vi "PUMP_main.vi"   [LabVIEW 2015]
uses:
  CONTROLS/Q_main_element.ctl
  CONTROLS/Q_PUMP_element.ctl
  <userlib>/Fluigent/Fluigent MFCS/FluigentMFCS_Full.llb/_EZmfcsRefNum.ctl
  <userlib>/Fluigent/Fluigent MFCS/FluigentMFCS_Full.llb/_EZmfcsEnum.ctl
  <userlib>/Fluigent/Fluigent FRP/FluigentFRP.llb/_frpEnum.ctl
  <userlib>/Fluigent/Fluigent MFCS/FluigentMFCS_Full.llb/_EZmfcsSN.ctl
  GLOBAL/Global_PUMP.vi
  GLOBAL/Global_ABORT.vi
  GLOBAL/Global_MAIN.vi
  <userlib>/Fluigent/Fluigent MFCS/FluigentMFCS_Full.llb/MFCS_EZ Initialization.vi
  <userlib>/Fluigent/Fluigent MFCS/FluigentMFCS_Full.llb/MFCS_EZ Close.vi
types:
  T1 = typedef "_frpRefNum" = refnum<k1>
  T2 = typedef "_EZmfcsRefNum.ctl" = refnum<k1>
  T3 = typedef "Q_PUMP_element.ctl" = cluster{"variant":variant, "Instruction":enum16{"PUMP_idle", "PUMP_initialize", "PUMP_error", "PUMP_security_stop", "PUMP_read_pressure", "PUMP_change_pressure", "PUMP_init_merFISH", "PUMP_change_presure_merFISH", "PUMP_zero_pressure_merFISH", "PUMP_close_merFISH", "PUMP_stop"}}
  T4 = typedef "Q_main_element.ctl" = cluster{"variant":variant, "Instruction":enum16{"Main_idle", "Main_initialize", "Main_initialize_TDMS", "Main_initialize_Queue", "Main_error", "Main_DAQ_initialization_results", "Main_ASI_initialization_results", "Main_Piezo_initialization_results", "Main_Valve_initialization_results", "Main_Pump_initialization_results", "Main_CAMERA_initialization_results", "Main_FPGA_initialization_results", "Main_DAQ_error", "Main_ASI_error", "Main_Piezo_error", "Main_CAMERA_error", "Main_Valve_error", "Main_Pump_error", "Main_FPGA_error", "Main_start_acquiring", "Main_not_acquiring", "Main_acquiring", "Main_stop_acquiring", "Main_change_exposure", "Main_change_z_scan_parameters", "Main_define_ROI", "Main_define_mosaic", "Main_read_kinetic_time", "Main_cooler", "Main_read_temperature", "Main_save_XY", "Main_load_XY", "Main_discard_XY", "Main_move_to_XY", "Main_measure_QPD", "Main_autofocus_calibration", "Main_autofocus_initialization", "Main_autofocus_stop", "Main_save_PID", "Main_change_H_valve_position", "Main_two_way_valve", "Main_save_movie", "Main_init_single_scan", "Main_single_scan", "Main_stop_single_scan", "Main_merFISH_illumination_parameters", "Main_merFISH_buffer_probe_list", "Main_merFISH_injections_procedure", "Main_merFISH_save_setpoint", "Main_merFISH_DAPI_parameters", "Main_merFISH_Brightfield_parameters", "Main_merFISH_save_embryo_ROI", "Main_merFISH_init", "Main_merFISH_resume", "Main_merFISH_start_autofocus", "Main_merFISH_open_close_valve_merFISH", "Main_merFISH_open_close_valve_photobleaching", "Main_merFISH_hybridization", "Main_merFISH_move_to_ROI", "Main_merFISH_wait_stabilization", "Main_merFISH_move_to_REF", "Main_merFISH_scan", "Main_merFISH_photobleaching_injection", "Main_merFISH_photobleaching", "Main_merFISH_send_email", "Main_merFISH_close", "Main_STOP"}}
  T5 = typedef "_EZmfcsSN.ctl" = u16
  T6 = cluster{"Pressure (mbar)":i32, "Volume (µl)":i32, "Flow rate (ul/min) ":i32}
  T7 = enum16{"PUMP_idle", "PUMP_initialize", "PUMP_error", "PUMP_security_stop", "PUMP_read_pressure", "PUMP_change_pressure", "PUMP_init_merFISH", "PUMP_change_presure_merFISH", "PUMP_zero_pressure_merFISH", "PUMP_close_merFISH", "PUMP_stop"}
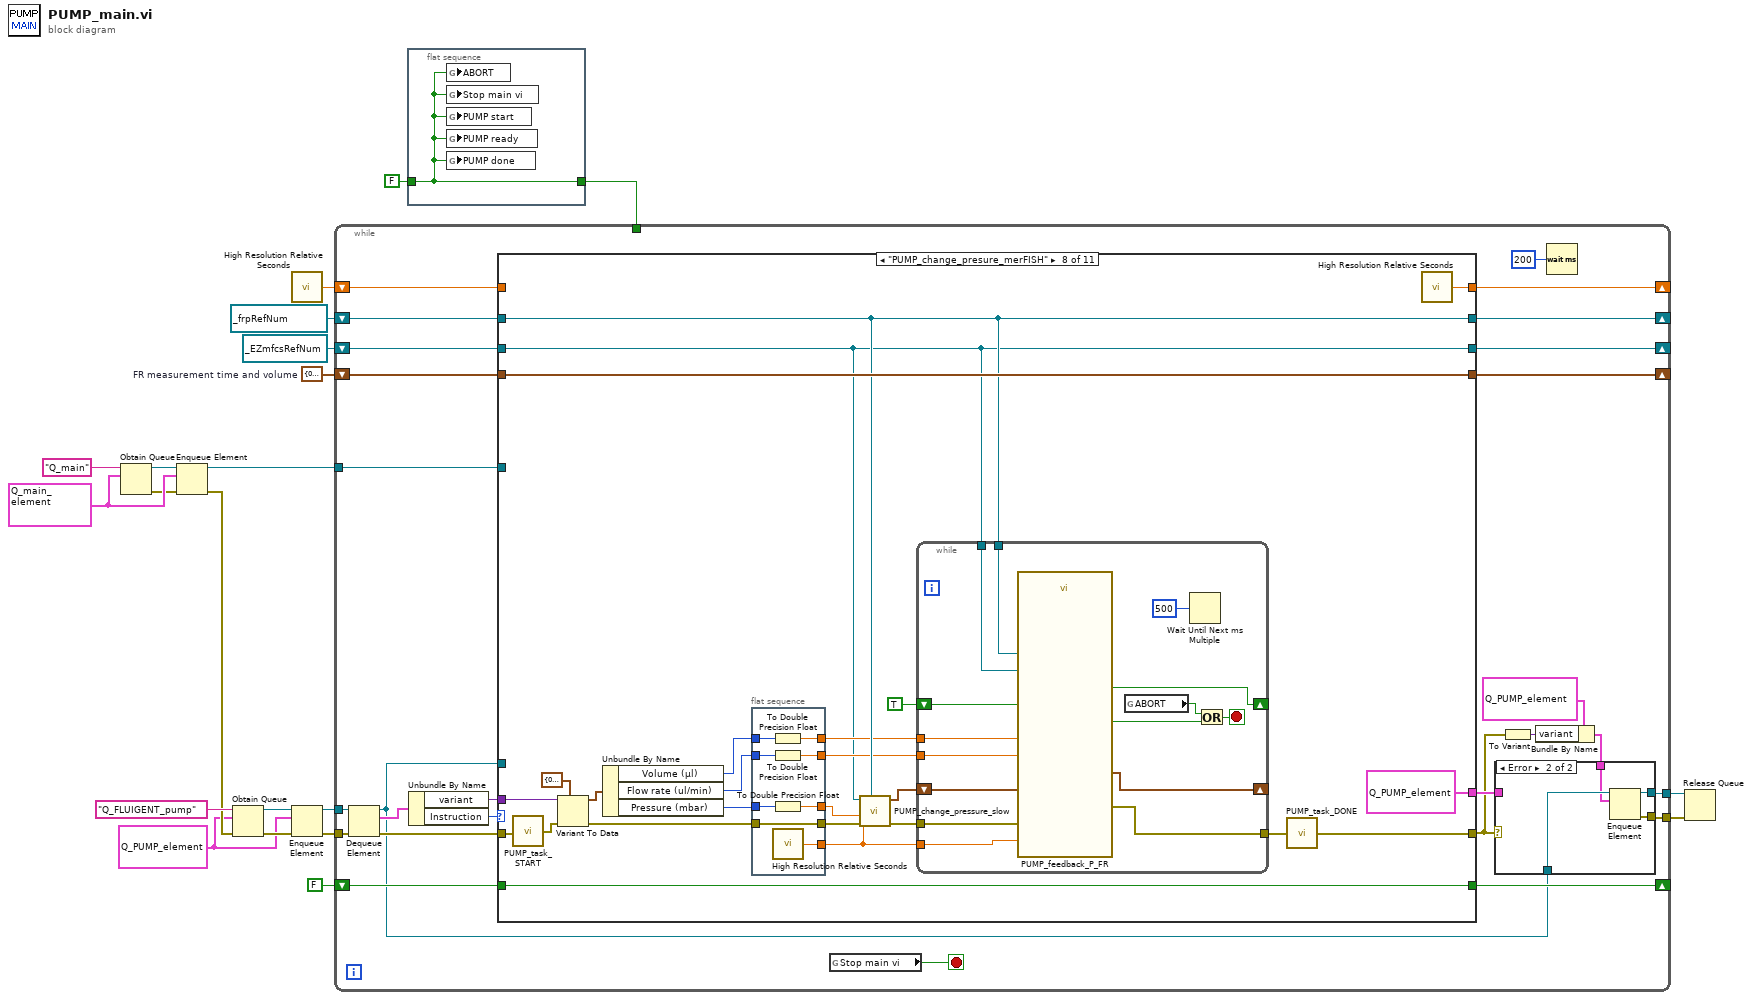
[diagram p0: block diagram]
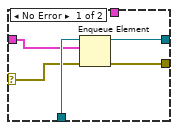
[diagram p2: hidden frame]
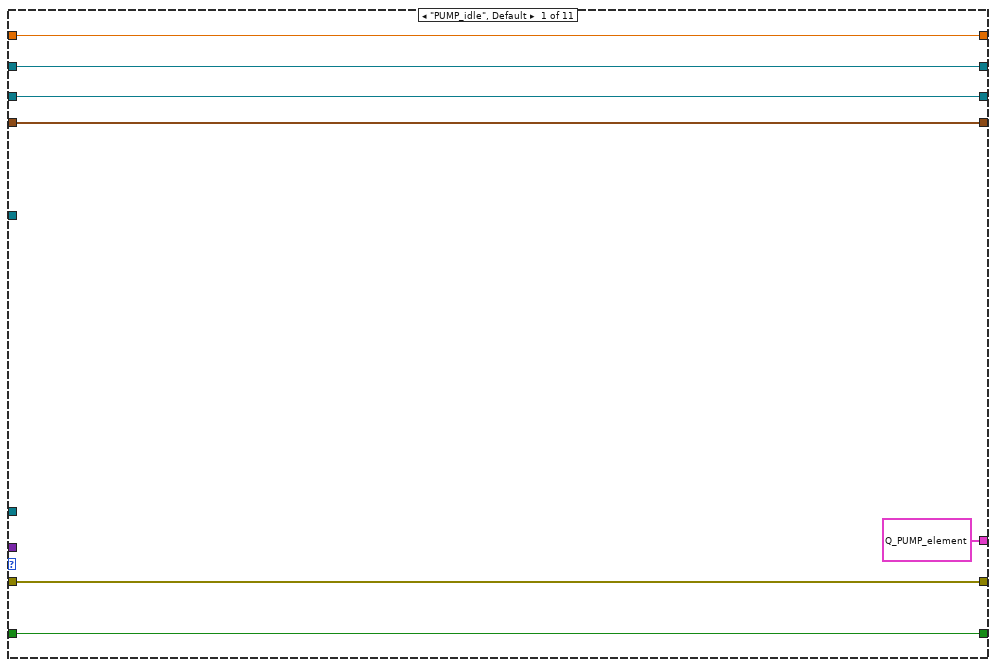
[diagram p3: hidden frame]
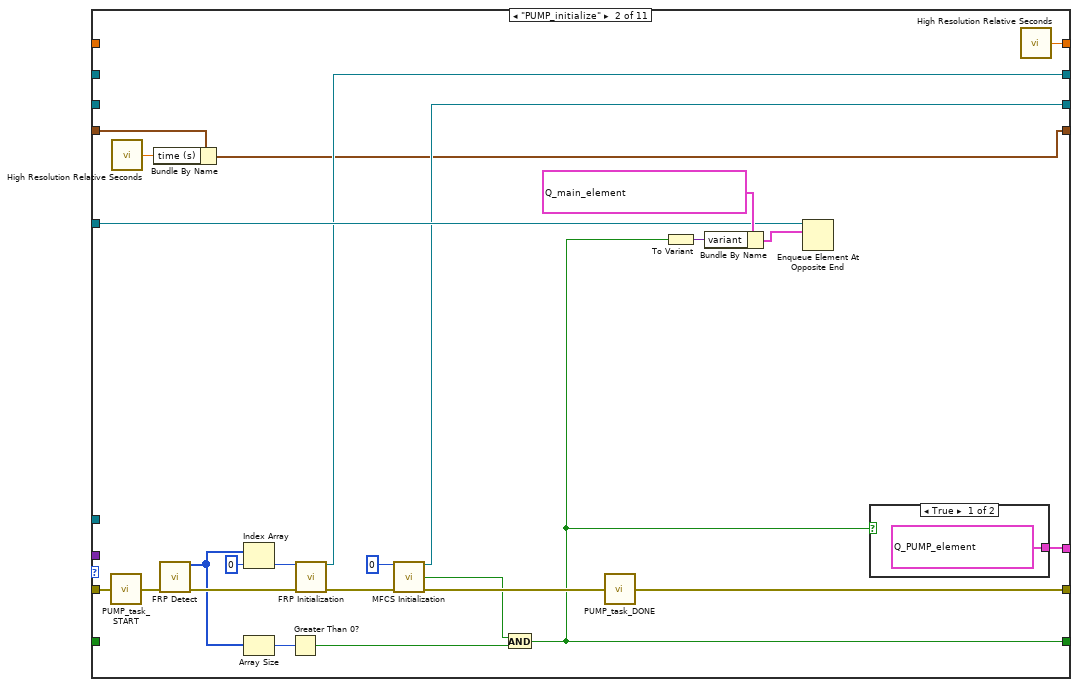
[diagram p4: hidden frame]
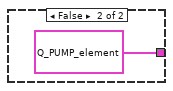
[diagram p5: hidden frame]
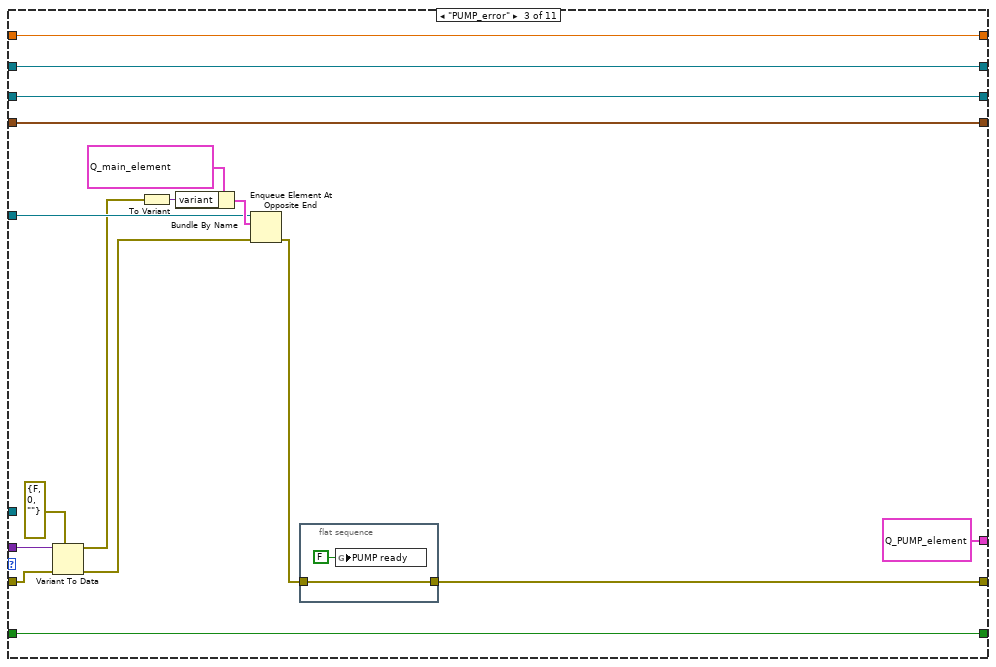
[diagram p6: hidden frame]
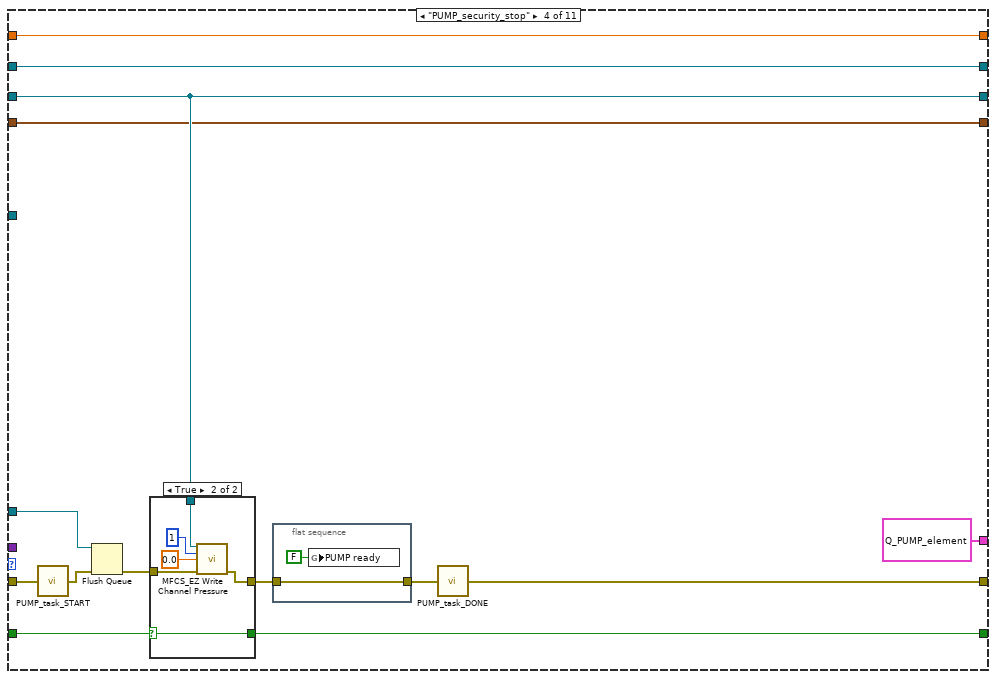
[diagram p7: hidden frame]
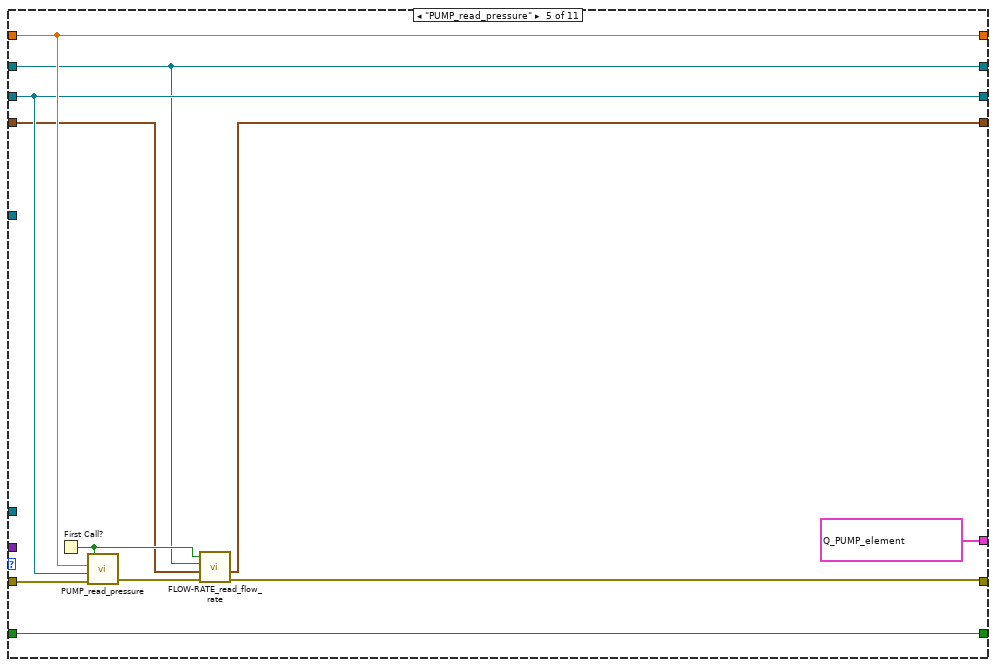
[diagram p9: hidden frame]
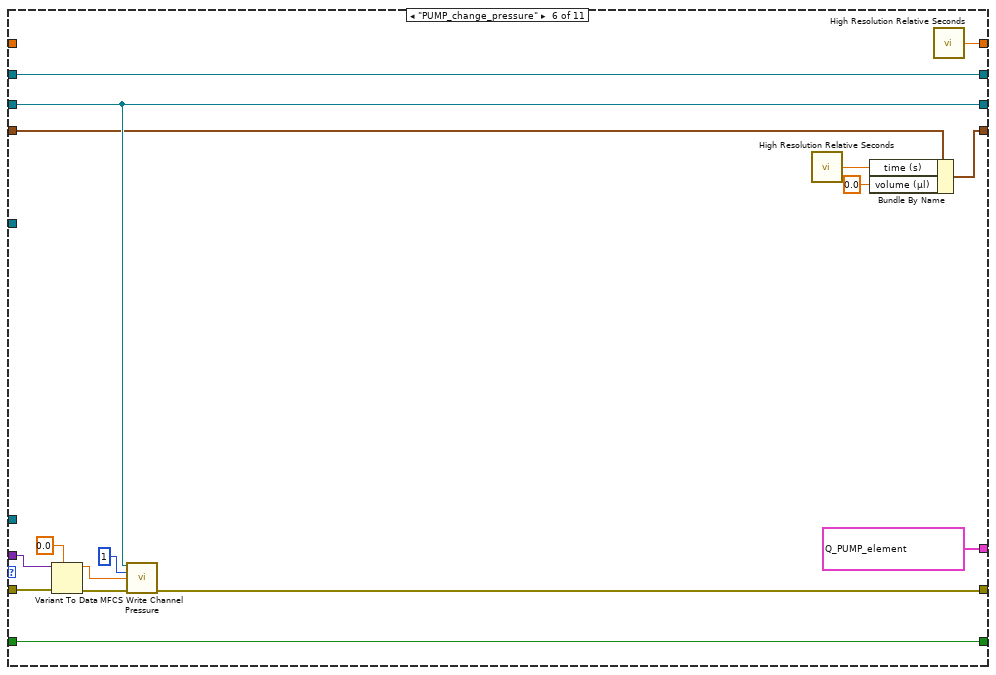
[diagram p10: hidden frame]
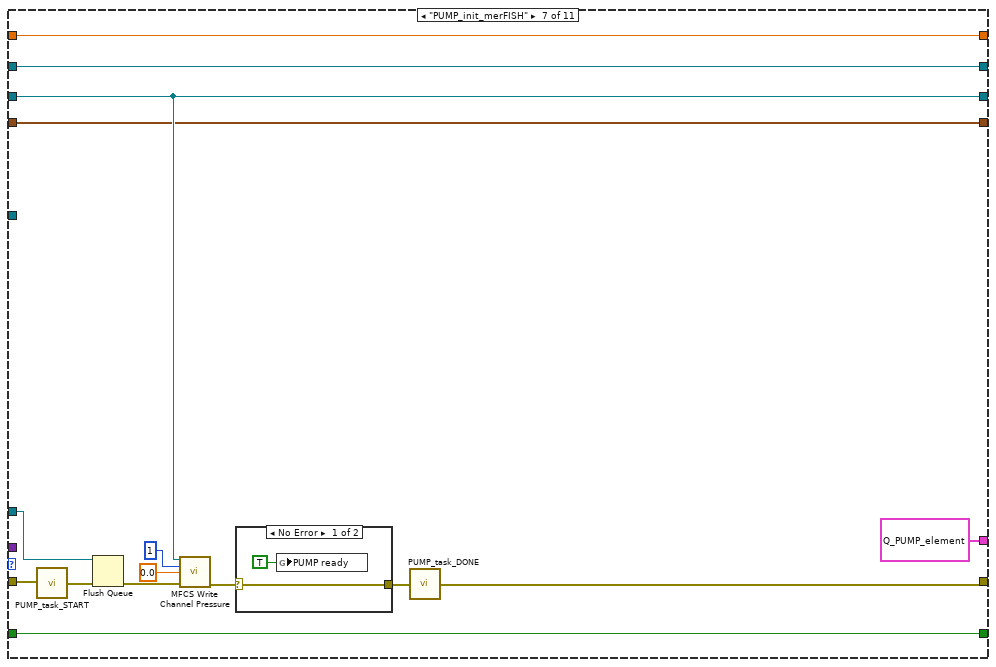
[diagram p11: hidden frame]
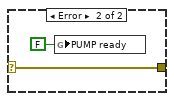
[diagram p12: hidden frame]
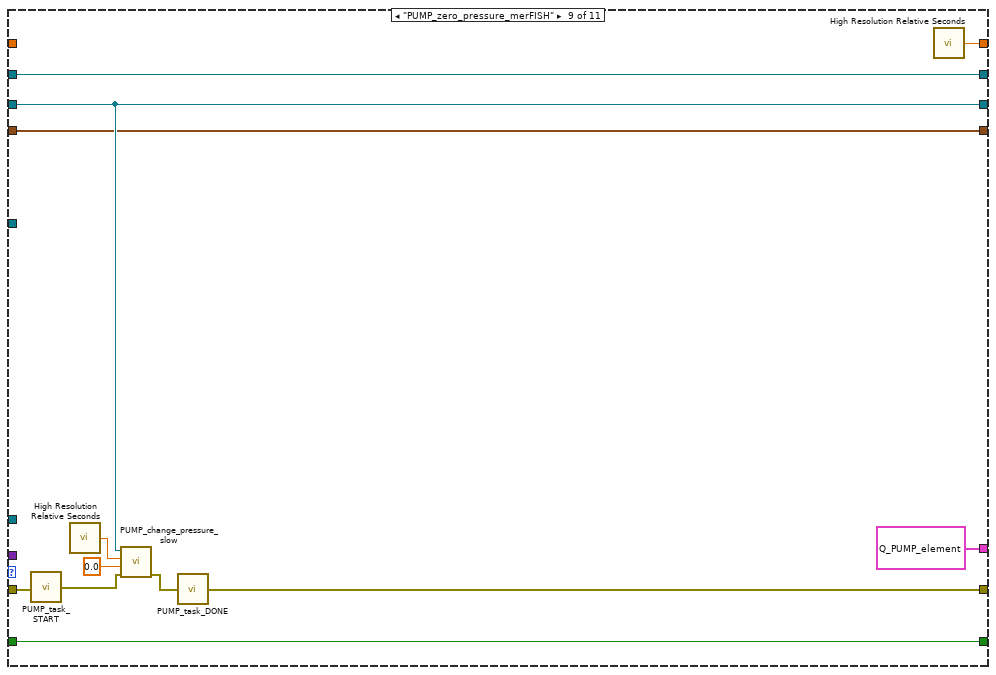
[diagram p13: hidden frame]
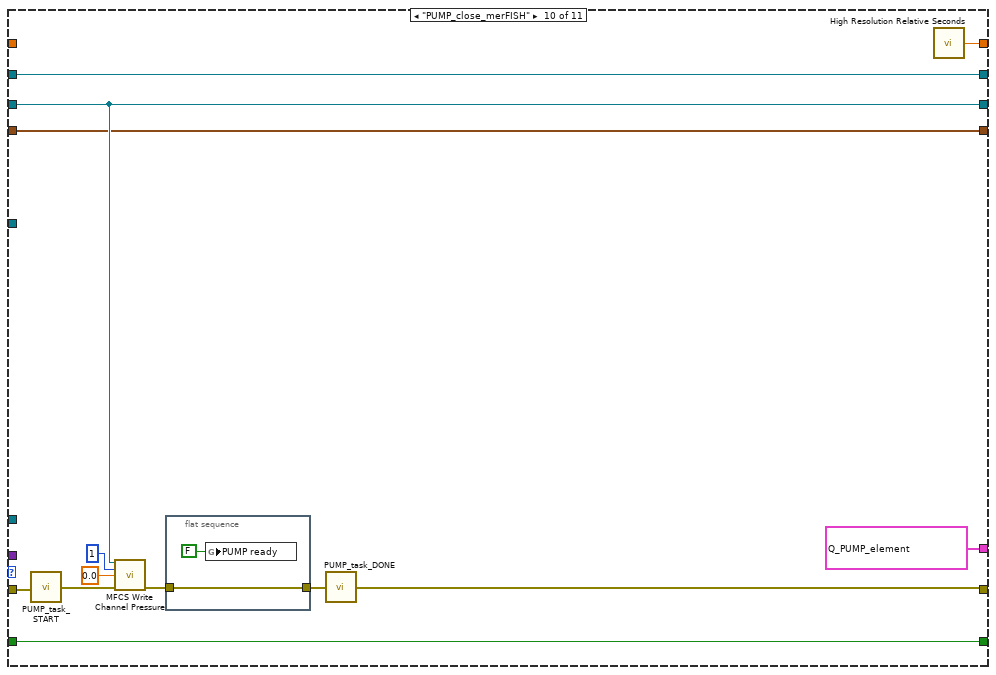
[diagram p14: hidden frame]
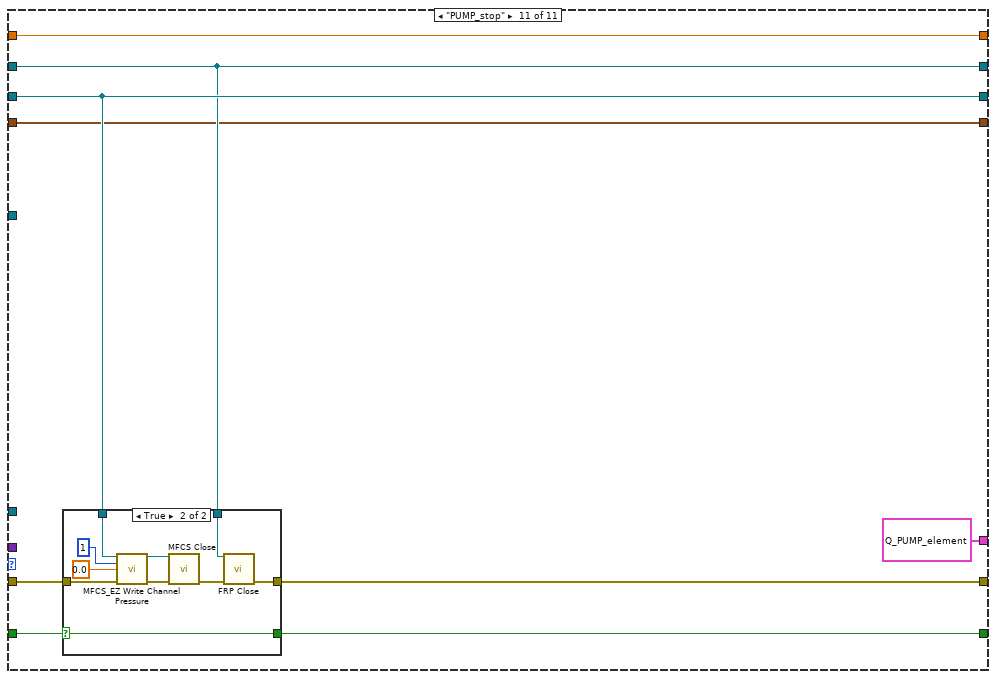
[diagram p15: hidden frame]
diagram:
  w1 = cluster{"time (s)":dbl, "volume (µl)":dbl} {"time (s)"=0.0, "volume (µl)"=0.0}  # FR measurement time and volume
  w2 = T1 refnum items=["fluigentFRP"] ("FRP out")
  w5 = T2 refnum items=["EZ_MFCS"] ("MFCS_EZ out")
  w6 = T3 {"variant"=variant, "Instruction"=enum."PUMP_idle"} ("Q_PUMP")
  w14 = T4 {"variant"=variant, "Instruction"=enum."Main_idle"} ("Q_main_element")
  n1 = Obtain Queue(name (unnamed)="Q_main", element data type=w14) -> (queue out=w12:refnum<queue>, error out=w13:errorcluster)  [unwired: 3 in, 1 out]
  n2 = Enqueue Element(queue=w12, element=w14, error in (no error)=w13) -> (queue out=w10:refnum<queue>, error out=w7:errorcluster)  [unwired: 1 in, 1 out]
  n3 = Obtain Queue(name (unnamed)="Q_FLUIGENT_pump", element data type=w6, error in (no error)=w7) -> (queue out=w20:refnum<queue>, error out=w19:errorcluster)  [unwired: 2 in, 1 out]
  n4 = call <vilib>:"High Resolution Relative Seconds.vi"() -> ("relative seconds"=w4:dbl)
  n5 = Enqueue Element(queue=w20, element=w6, error in (no error)=w19) -> (queue out=w18:refnum<queue>, error out=w17:errorcluster)  [unwired: 1 in, 1 out]
  n6 = while {
    tunnel: w18 -> [w47]
    tunnel: w17 -> [w46]
    tunnel: [w41] -> w16
    tunnel: [w40] -> w15
    tunnel: w10 -> [w39]
    tunnel: w8 -> [_]
    shift-right: [w32] -> _
    shift-left: w5 -> [w31]
    shift-right: [w30] -> _
    shift-left: w4 -> [w29]
    shift-right: [w27] -> _
    shift-left: FALSE -> [w28]
    shift-right: [w25] -> _
    shift-left: w2 -> [w26]
    shift-right: [w23] -> _
    shift-left: w1 -> [w24]
    stop <- w48 stop-if-true
    n7 = Dequeue Element(queue=w47, error in (no error)=w46) -> (queue out=w22:refnum<queue>, element=w45:T3, error out=w43:errorcluster)  [unwired: 1 in, 1 out]
    n8 = Unbundle By Name(w45) -> ("variant"=w38:variant, "Instruction"=w44:T7)
    n9 = case shown="\"PUMP_change_presure_merFISH\"" w44 {
      tunnel: w43 -> [w64 w89 w101 w123 w144 w161 w174 w201 w238 w251 w262]
      tunnel: [w64 w69 w94 w118 w140 w150 w172 w197 w237 w250 w263] -> w35
      tunnel: [T3 {"variant"=variant, "Instruction"=enum."PUMP_idle"} ("Q_PUMP") w82 T3 {"variant"=variant, "Instruction"=enum."PUMP_idle"} ("Q_PUMP") T3 {"variant"=variant, "Instruction"=enum."PUMP_idle"} ("Q_PUMP") T3 {"variant"=variant, "Instruction"=enum."PUMP_read_pressure"} ("Q_PUMP") T3 {"variant"=variant, "Instruction"=enum."PUMP_read_pressure"} ("Q_PUMP") T3 {"variant"=variant, "Instruction"=enum."PUMP_idle"} ("Q_PUMP") T3 {"variant"=variant, "Instruction"=enum."PUMP_idle"} ("Q_PUMP") T3 {"variant"=variant, "Instruction"=enum."PUMP_idle"} ("Q_PUMP") T3 {"variant"=variant, "Instruction"=enum."PUMP_read_pressure"} ("Q_PUMP") T3 {"variant"=variant, "Instruction"=enum."PUMP_idle"} ("Q_PUMP")] -> w42
      tunnel: w39 -> [_ w84 w103 _ _ _ _ _ _ _ _]
      tunnel: w38 -> [_ _ w100 _ _ w160 _ w205 _ _ _]
      tunnel: w22 -> [_ _ _ w121 _ _ w167 _ _ _ _]
      tunnel: [w62 w83 w107 w119 w138 w152 w164 w183 w236 w244 w261] -> w32
      tunnel: w31 -> [w62 _ w107 w119 w138 w152 w164 w183 w236 w244 w261]
      tunnel: [w61 w81 w97 w117 w143 w154 w176 w203 w239 w252 w260] -> w30
      tunnel: w29 -> [w61 _ w97 w117 w143 _ w176 _ _ _ w260]
      tunnel: w28 -> [w60 _ w96 w116 w142 w153 w165 w202 w235 w249 w259]
      tunnel: [w60 w70 w96 w115 w142 w153 w165 w202 w235 w249 w258] -> w27
      tunnel: w26 -> [w59 _ w93 w112 w137 w151 w163 w189 w230 w242 w257]
      tunnel: [w59 w68 w93 w112 w137 w151 w163 w189 w230 w242 w257] -> w25
      tunnel: w24 -> [w58 w67 w92 w111 w136 w149 w162 w193 w229 w241 w256]
      tunnel: [w58 w65 w92 w111 w135 w146 w162 w193 w229 w241 w256] -> w23
      frame "PUMP_idle", Default {
      }
      frame "PUMP_initialize" {
        n10 = call "PUMP_task_START.vi"("error in"=w89) -> ("error out"=w79:errorcluster)
        n11 = call <vilib>:"High Resolution Relative Seconds.vi"() -> ("relative seconds"=w66:dbl)
        n12 = Bundle By Name(cluster=w67, "time (s)"=w66) -> (w65:cluster{"time (s)":dbl, "volume (µl)":dbl})
        n13 = call <userlib>:"FRP Detect.vi"("error in (no error)"=w79) -> ("FLOWBOARD List"=w74:u16[], "error out"=w78:errorcluster)  [unwired: 13 in]
        n14 = Index Array(array=w74, index=0) -> (element=w76:u16)
        n15 = Array Size(array=w74) -> (size(s)=w73:i32)
        n16 = Greater Than 0?(x=w73) -> (x > 0?=w72:bool)
        n17 = call <userlib>:"FRP Initialization.vi"("Serial Number"=w76, "error in (no error)"=w78) -> ("FRP out"=w68:T1, "error out"=w75:errorcluster)  [unwired: 11 in, 1 out]
        n18 = call-poly <userlib>:"MFCS Initialization.vi"("SN MFCS_EZ"=T5 0, "error in (no error)"=w75) -> ("MFCS_EZ"=w83:T2, "MFCS Found (TF)"=w71:bool, "error out"=w80:errorcluster)  [unwired: 11 in]
        n19 = And(x=w71, y=w72) -> (x .and. y?=w70:bool)
        n20 = call "PUMP_task_DONE.vi"("error in"=w80) -> ("error out"=w69:errorcluster)
        n21 = To Variant(anything=w70) -> (Variant=w86:variant)
        n22 = Bundle By Name(cluster=T4 {"variant"=variant, "Instruction"=enum."Main_Pump_initialization_results"} ("element"), "variant"=w86) -> (w87:T4)
        n23 = Enqueue Element At Opposite End(queue=w84, element=w87) -> ()  [unwired: 2 in, 3 out]
        n24 = case shown="True" w70 {
          tunnel: [T3 {"variant"=variant, "Instruction"=enum."PUMP_read_pressure"} ("Q_PUMP") T3 {"variant"=variant, "Instruction"=enum."PUMP_idle"} ("Q_PUMP")] -> w82
          frame True {
          }
          frame False {
          }
        }
        n25 = call <vilib>:"High Resolution Relative Seconds.vi"() -> ("relative seconds"=w81:dbl)
      }
      frame "PUMP_error" {
        n26 = Variant To Data(error in=w101, type=errorcluster {"status"=FALSE, "code"=0, "source"=""} ("error out"), Variant=w100) -> (data=w99:errorcluster, error out=w98:errorcluster)
        n27 = To Variant(anything=w99) -> (Variant=w105:variant)
        n28 = Bundle By Name(cluster=T4 {"variant"=variant, "Instruction"=enum."Main_Pump_error"} ("Q_main_element"), "variant"=w105) -> (w106:T4)
        n29 = Enqueue Element At Opposite End(queue=w103, element=w106, error in (no error)=w98) -> (error out=w95:errorcluster)  [unwired: 1 in, 2 out]
        n30 = flat-sequence {
          tunnel: w95 -> [w110]
          tunnel: [w110] -> w94
          frame #0 {
            n31 = global write "Global_PUMP.vi" "PUMP ready"(FALSE ("PUMP ready")) -> ()
          }
        }
      }
      frame "PUMP_security_stop" {
        n32 = call "PUMP_task_START.vi"("error in"=w123) -> ("error out"=w122:errorcluster)
        n33 = Flush Queue(queue=w121, error in (no error)=w122) -> (error out=w120:errorcluster)  [unwired: 2 out]
        n34 = case shown="True" w116 {
          selector: w116 -> [w127 w129]
          tunnel: w120 -> [w128 w132]
          tunnel: w119 -> [_ w131]
          tunnel: [w128 w130] -> w114
          tunnel: [w127 w129] -> w115
          frame False {
          }
          frame True {
            n35 = call <userlib>:"MFCS_EZ Write Channel Pressure.vi"("MFCS_EZ"=w131, "Channel Number (default=1)"=u8 1, "Pressure (mBar)"=0.0, "error in (no error)"=w132) -> ("error out"=w130:errorcluster)  [unwired: 10 in, 1 out]
          }
        }
        n36 = flat-sequence {
          tunnel: w114 -> [w126]
          tunnel: [w126] -> w113
          frame #0 {
            n37 = global write "Global_PUMP.vi" "PUMP ready"(FALSE ("PUMP ready")) -> ()
          }
        }
        n38 = call "PUMP_task_DONE.vi"("error in"=w113) -> ("error out"=w118:errorcluster)
      }
      frame "PUMP_read_pressure" {
        n39 = First Call?() -> (First Call?: T/F=w139:bool)
        n40 = call "PUMP_read_pressure.vi"("error in"=w144, "MFCS_EZ"=w138, "t0"=w143, "Reset"=w139) -> ("error out"=w141:errorcluster)  [unwired: 2 out]
        n41 = call "FLOW-RATE_read_flow_rate.vi"("error in"=w141, "Data t i-1"=w136, "FRP out"=w137, "Reset"=w139) -> ("error out"=w140:errorcluster, "Data t i"=w135:cluster{"time (s)":dbl, "volume (µl)":dbl})  [unwired: 2 out]
      }
      frame "PUMP_change_pressure" {
        n42 = Variant To Data(error in=w161, type=0.0 ("Pressure (mbar)"), Variant=w160) -> (data=w156:dbl, error out=w157:errorcluster)
        n43 = call-poly <userlib>:"MFCS Write Channel Pressure.vi"("MFCS_EZ"=w152, "Channel Number (default=1)"=u8 1, "Pressure (mBar)"=w156, "error in (no error)"=w157) -> ("error out"=w150:errorcluster)  [unwired: 10 in, 1 out]
        n44 = call <vilib>:"High Resolution Relative Seconds.vi"() -> ("relative seconds"=w148:dbl)
        n45 = Bundle By Name(cluster=w149, "time (s)"=w148, "volume (µl)"=0.0) -> (w146:cluster{"time (s)":dbl, "volume (µl)":dbl})
        n46 = call <vilib>:"High Resolution Relative Seconds.vi"() -> ("relative seconds"=w154:dbl)
      }
      frame "PUMP_init_merFISH" {
        n47 = call "PUMP_task_START.vi"("error in"=w174) -> ("error out"=w168:errorcluster)
        n48 = Flush Queue(queue=w167, error in (no error)=w168) -> (error out=w166:errorcluster)  [unwired: 2 out]
        n49 = call-poly <userlib>:"MFCS Write Channel Pressure.vi"("MFCS_EZ"=w164, "Channel Number (default=1)"=u8 1, "Pressure (mBar)"=0.0, "error in (no error)"=w166) -> ("error out"=w171:errorcluster)  [unwired: 10 in, 1 out]
        n50 = case shown="No Error" w171 {
          selector: w171 -> [w178 w180]
          tunnel: [w178 w180] -> w170
          frame No Error {
            n51 = global write "Global_PUMP.vi" "PUMP ready"(TRUE ("PUMP ready")) -> ()
          }
          frame Error {
            n52 = global write "Global_PUMP.vi" "PUMP ready"(FALSE ("PUMP ready")) -> ()
          }
        }
        n53 = call "PUMP_task_DONE.vi"("error in"=w170) -> ("error out"=w172:errorcluster)
      }
      frame "PUMP_change_presure_merFISH" {
        n54 = call "PUMP_task_START.vi"("error in"=w201) -> ("error out"=w200:errorcluster)
        n55 = Variant To Data(error in=w200, type=T6 {"Pressure (mbar)"=0, "Volume (µl)"=0, "Flow rate (ul/min) "=0} ("input data cluster"), Variant=w205) -> (data=w188:T6, error out=w199:errorcluster)
        n56 = Unbundle By Name(w188) -> ("Volume (µl)"=w185:i32, "Flow rate (ul/min)"=w187:i32, "Pressure (mbar)"=w198:i32)
        n57 = flat-sequence {
          tunnel: w199 -> [w228]
          tunnel: [w228] -> w196
          tunnel: [w227] -> w191
          tunnel: w198 -> [w226]
          tunnel: [w225] -> w194
          tunnel: [w223] -> w186
          tunnel: w187 -> [w224]
          tunnel: w185 -> [w222]
          tunnel: [w221] -> w184
          frame #0 {
            n58 = To Double Precision Float(number=w222) -> (double precision float=w221:dbl)
            n59 = To Double Precision Float(number=w224) -> (double precision float=w223:dbl)
            n60 = To Double Precision Float(number=w226) -> (double precision float=w225:dbl)
            n61 = call <vilib>:"High Resolution Relative Seconds.vi"() -> ("relative seconds"=w227:dbl)
          }
        }
        n62 = call "PUMP_change_pressure_slow.vi"("FRP out"=w189, "error in"=w196, "Pressure setpoint"=w194, "t0"=w191, "MFCS_EZ"=w183) -> ("error out"=w195:errorcluster, "FR Data"=w190:cluster{"time (s)":dbl, "volume (µl)":dbl})  [unwired: 2 in]
        n63 = while {
          tunnel: w195 -> [w217]
          tunnel: w191 -> [w208]
          shift-right: [w211] -> _
          shift-left: w190 -> [w212]
          tunnel: w189 -> [w215]
          tunnel: w184 -> [w213]
          tunnel: w186 -> [w209]
          tunnel: w183 -> [w214]
          tunnel: [w216] -> w182
          shift-right: [w206] -> _
          shift-left: TRUE -> [w207]
          stop <- w219 stop-if-true
          n64 = call "PUMP_feedback_P_FR.vi"("Allow email"=w207, "FR Data"=w212, "t0"=w208, "FRP"=w215, "error in"=w217, "MFCS_EZ"=w214, "Volume setpoint"=w213, "FR setpoint"=w209) -> ("error out"=w216:errorcluster, "Allow email out"=w206:bool, "FR Data OUT"=w211:cluster{"time (s)":dbl, "volume (µl)":dbl}, "volume reached?"=w210:bool)
          n65 = global read "Global_ABORT.vi" "ABORT"() -> (w218:bool)
          n66 = Wait Until Next ms Multiple(millisecond multiple=u32 500) -> ()  [unwired: 1 out]
          n67 = Or(x=w218, y=w210) -> (x .or. y?=w219:bool)
        }
        n68 = call "PUMP_task_DONE.vi"("error in"=w182) -> ("error out"=w197:errorcluster)
        n69 = call <vilib>:"High Resolution Relative Seconds.vi"() -> ("relative seconds"=w203:dbl)
      }
      frame "PUMP_zero_pressure_merFISH" {
        n70 = call "PUMP_task_START.vi"("error in"=w238) -> ("error out"=w234:errorcluster)
        n71 = call <vilib>:"High Resolution Relative Seconds.vi"() -> ("relative seconds"=w231:dbl)
        n72 = call "PUMP_change_pressure_slow.vi"("error in"=w234, "Pressure setpoint"=0.0, "t0"=w231, "MFCS_EZ"=w236) -> ("error out"=w232:errorcluster)  [unwired: 3 in, 1 out]
        n73 = call "PUMP_task_DONE.vi"("error in"=w232) -> ("error out"=w237:errorcluster)
        n74 = call <vilib>:"High Resolution Relative Seconds.vi"() -> ("relative seconds"=w239:dbl)
      }
      frame "PUMP_close_merFISH" {
        n75 = call "PUMP_task_START.vi"("error in"=w251) -> ("error out"=w246:errorcluster)
        n76 = call-poly <userlib>:"MFCS Write Channel Pressure.vi"("MFCS_EZ"=w244, "Channel Number (default=1)"=u8 1, "Pressure (mBar)"=0.0, "error in (no error)"=w246) -> ("error out"=w245:errorcluster)  [unwired: 10 in, 1 out]
        n77 = flat-sequence {
          tunnel: [w254] -> w248
          tunnel: w245 -> [w254]
          frame #0 {
            n78 = global write "Global_PUMP.vi" "PUMP ready"(FALSE ("PUMP ready")) -> ()
          }
        }
        n79 = call "PUMP_task_DONE.vi"("error in"=w248) -> ("error out"=w250:errorcluster)
        n80 = call <vilib>:"High Resolution Relative Seconds.vi"() -> ("relative seconds"=w252:dbl)
      }
      frame "PUMP_stop" {
        n81 = case shown="True" w259 {
          selector: w259 -> [w265 w270]
          tunnel: [w266 w267] -> w263
          tunnel: w262 -> [w266 w275]
          tunnel: w261 -> [_ w272]
          tunnel: [w265 w270] -> w258
          tunnel: w257 -> [_ w268]
          frame False {
          }
          frame True {
            n82 = call <userlib>:"MFCS_EZ Write Channel Pressure.vi"("MFCS_EZ"=w272, "Channel Number (default=1)"=u8 1, "Pressure (mBar)"=0.0, "error in (no error)"=w275) -> ("error out"=w274:errorcluster)  [unwired: 10 in, 1 out]
            n83 = call-poly <userlib>:"MFCS Close.vi"("MFCS_EZ"=w272, "error in (no error)"=w274) -> ("error out"=w269:errorcluster)  [unwired: 13 in]
            n84 = call <userlib>:"FRP Close.vi"("FRP"=w268, "error in (no error)"=w269) -> ("error out"=w267:errorcluster)  [unwired: 13 in]
          }
        }
      }
    }
    n85 = global read "Global_MAIN.vi" "Stop main vi"() -> (w48:bool)
    n86 = To Variant(anything=w35) -> (Variant=w36:variant)
    n87 = Bundle By Name(cluster=T3 {"variant"=variant, "Instruction"=enum."PUMP_error"} ("Q_PUMP"), "variant"=w36) -> (w37:T3)
    n88 = case shown="Error" w35 {
      selector: w35 -> [w50 _]
      tunnel: w42 -> [w49 _]
      tunnel: [w53 w57] -> w41
      tunnel: [w52 w56] -> w40
      tunnel: w22 -> [w51 w55]
      tunnel: w37 -> [_ w54]
      frame No Error {
        n89 = Enqueue Element(queue=w51, element=w49, error in (no error)=w50) -> (queue out=w53:refnum<queue>, error out=w52:errorcluster)  [unwired: 1 in, 1 out]
      }
      frame Error {
        n90 = Enqueue Element(queue=w55, element=w54) -> (queue out=w57:refnum<queue>, error out=w56:errorcluster)  [unwired: 2 in, 1 out]
      }
    }
    n91 = Wait (ms)(milliseconds to wait=u32 200) -> ()  [unwired: 1 out]
  }
  n92 = flat-sequence {
    tunnel: FALSE ("Stop main vi") -> [w276]
    tunnel: [w276] -> w8
    frame #0 {
      n93 = global write "Global_ABORT.vi" "ABORT"(w276) -> ()
      n94 = global write "Global_MAIN.vi" "Stop main vi"(w276) -> ()
      n95 = global write "Global_PUMP.vi" "PUMP start"(w276) -> ()
      n96 = global write "Global_PUMP.vi" "PUMP ready"(w276) -> ()
      n97 = global write "Global_PUMP.vi" "PUMP done"(w276) -> ()
    }
  }
  n98 = Release Queue(queue=w16, error in (no error)=w15) -> ()  [unwired: 1 in, 3 out]
